vi "3-1.vi"() -> ()   [LabVIEW 2019, in "3.lvlib"]
uses:
  3.lvlib
  <vilib>/Utility/file.llb/Read Delimited Spreadsheet (string).vi
panel:
  out "power consumption":u32
  out "epsilon":u32
  out "gamma":u32
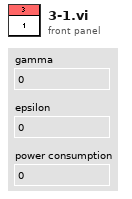
[diagram p1: front panel]
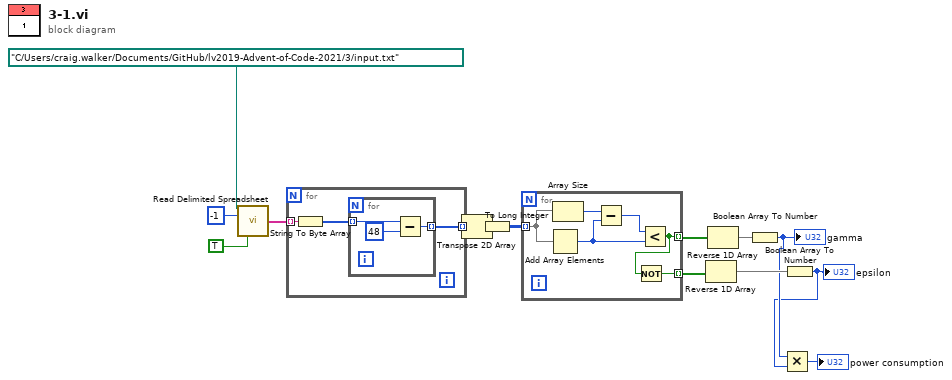
[diagram p0: block diagram]
diagram:
  n1 = call-poly <vilib>:"Read Delimited Spreadsheet.vi"("file path (dialog if empty)"=path "C:/Users/craig.walker/Documents/GitHub/lv2019-Advent-of-Code-2021/3/input.txt", "number of rows (all:-1)"=-1, "transpose? (F)"=TRUE) -> ("first row"=w10:string[])  [unwired: 7 in, 5 out]
  n2 = for {
    tunnel: w10 -> [w17] mode=indexing
    tunnel: [w15] -> w3 mode=indexing
    n3 = String To Byte Array(string=w17) -> (unsigned byte array=w16:u8[])
    n4 = for {
      tunnel: w16 -> [w20] mode=indexing
      tunnel: [w18] -> w15 mode=indexing
      n5 = Subtract(x=w20, y=u8 48) -> (x-y=w18:u8)
    }
  }
  n6 = Transpose 2D Array(2D array=w3) -> (transposed array=w1:u8[][])
  n7 = To Long Integer(number=w1) -> (32bit integer=w2:i32[][])
  n8 = for {
    tunnel: w2 -> [w26] mode=indexing
    tunnel: [w22] -> w11 mode=indexing
    tunnel: [w21] -> w8 mode=indexing
    n9 = Add Array Elements(numeric array=w26) -> (sum=w23:i32)
    n10 = Array Size(array=w26) -> (size(s)=w25:i32)
    n11 = Subtract(x=w25, y=w23) -> (x-y=w24:i32)
    n12 = Less?(x=w24, y=w23) -> (x < y?=w22:bool)
    n13 = Not(x=w22) -> (.not. x?=w21:bool)
  }
  n14 = Reverse 1D Array(array=w8) -> (reversed array=w7:bool[])
  n15 = Reverse 1D Array(array=w11) -> (reversed array=w9:bool[])
  n16 = Boolean Array To Number(Boolean array=w9) -> (number=w5:u32)
  "gamma" <- w5
  n17 = Boolean Array To Number(Boolean array=w7) -> (number=w4:u32)
  "epsilon" <- w4
  n18 = Multiply(x=w5, y=w4) -> (x*y=→"power consumption":u32)
